vi "GUI.Button.Disabled.vi"(8 "error in (no error)":errorcluster, 10 "buttonDisabled":T1(ring), 11 "buttonName":string) -> (0 "error out":errorcluster)   [LabVIEW 2019]
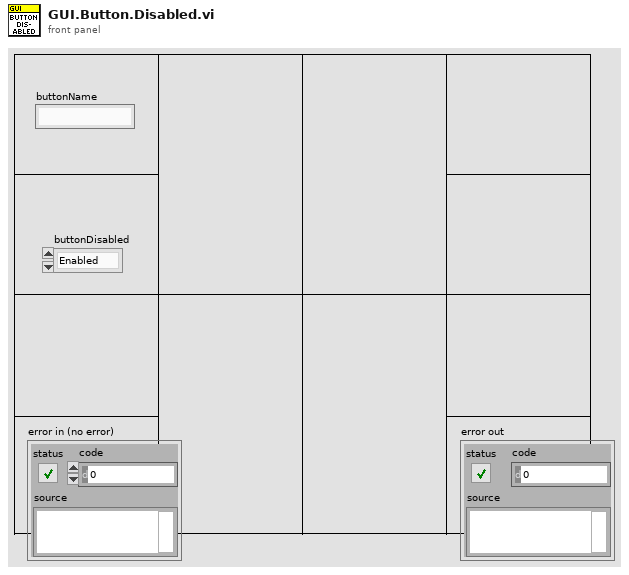
[diagram p1: front panel]
types:
  T1 = enum8{"Enabled", "Disabled", "Disabled and Grayed Out"}
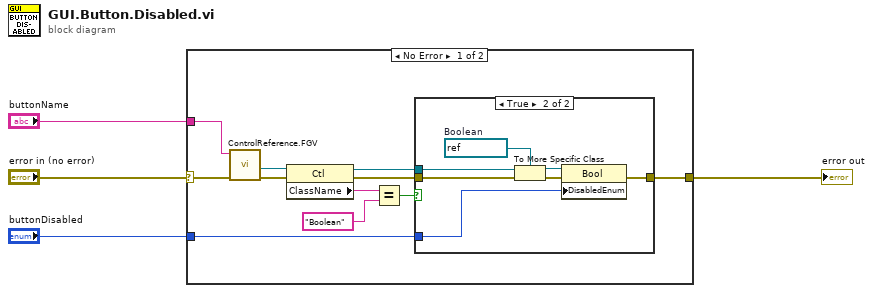
[diagram p0: block diagram]
diagram:
  n1 = case shown="No Error" "error in (no error)" {
    selector: "error in (no error)" -> [w14 w24]
    tunnel: [w15 w24] -> w3
    tunnel: "buttonName" -> [w13 _]
    tunnel: "buttonDisabled" -> [w5 _]
    frame No Error {
      n2 = call "ControlReference.FGV.vi"("error in (no error)"=w14, "controlLabelText"=w13) -> ("error out"=w12:errorcluster, "referenceToControl"=w10:refnum<vi>)  [unwired: 8 in]
      n3 = property class="Ctl"(reference=w10, error in=w12) -> (reference out=w6:refnum<vi>, error out=w11:errorcluster, "ClassName"=w9:string)
      n4 = Equal?(x=w9, y="Boolean") -> (x = y?=w7:bool)
      n5 = case shown="True" w7 {
        tunnel: w11 -> [w16 w19]
        tunnel: [w16 w20] -> w15
        tunnel: w6 -> [_ w18]
        tunnel: w5 -> [_ w17]
        frame False {
        }
        frame True {
          w22 = refnum<vi> refnum  # Boolean
          n6 = To More Specific Class(target class=w22, reference=w18, error in=w19) -> (specific class reference=w21:refnum<vi>, error out=w23:errorcluster)
          n7 = property class="Bool"(reference=w21, error in=w23, "DisabledEnum"=w17) -> (error out=w20:errorcluster)  [unwired: 1 out]
        }
      }
    }
    frame Error {
    }
  }
  "error out" <- w3
